vi "helperLoop.vi"(8 "error in (no error)":errorcluster, 11 "Connection Handler in":refnum<class "Connection Handler.lvclass">) -> (0 "error out":errorcluster, 3 "Connection Handler out":refnum<class "Connection Handler.lvclass">)   [LabVIEW 2017, in "Connection Handler.lvlib" / "Connection Handler.lvclass"]
uses:
  Connection Handler.lvclass
  Applications/National Instruments/LabVIEW 2017 64-bit/vi.lib/ActorFramework/Actor/Actor.lvclass
  Volumes/Data/Users/benji667/Git/BuildFarm/WebSocket Server/Actors/Actor wHelper/Actor wHelper/Actor wHelper.lvclass
  <vilib>/ActorFramework/Actor/Actor.lvclass/Actor.ctl
  <vilib>/ActorFramework/Message Enqueuer/Message Enqueuer.lvclass/Message Enqueuer.ctl
  Connection Handler.lvclass/Connection Handler.ctl
  Actor wHelper/Actor wHelper/Actor wHelper.lvclass/Actor wHelper.ctl
  Connection Handler Messages/Message Recieved Msg/Message Recieved Msg.lvclass/Message Recieved Msg.ctl
  Actor wHelper/Actor wHelper/Read StopHelperLoop Reg Ref.vi
  <vilib>/ActorFramework/Message Enqueuer/Init from Existing Queue.vi
  <vilib>/ActorFramework/Message Enqueuer/Enqueue.vi
  Connection Handler Messages/Message Recieved Msg/Message Recieved Msg.lvclass
  Applications/National Instruments/LabVIEW 2017 64-bit/vi.lib/ActorFramework/Message/Message.lvclass
  <vilib>/ActorFramework/Stop Msg/Stop Msg.lvclass
  <vilib>/ActorFramework/Message Priority Queue/Priority Enqueue.vi
  <vilib>/ActorFramework/Message Enqueuer/Message Enqueuer.lvclass
  Actor wHelper/Actor wHelper/Actor wHelper.lvclass
  <vilib>/MediaMongrels Ltd/WebSockets/Sockets/Socket/Socket.lvclass
  <vilib>/ActorFramework/Actor/Actor.lvclass
panel:
  out "Data":string
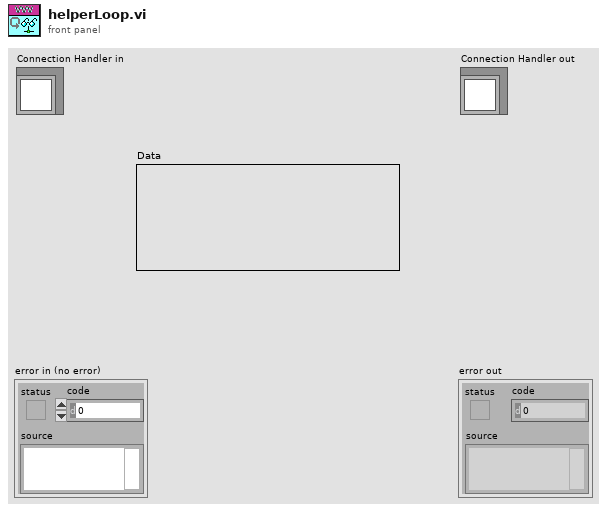
[diagram p1: front panel]
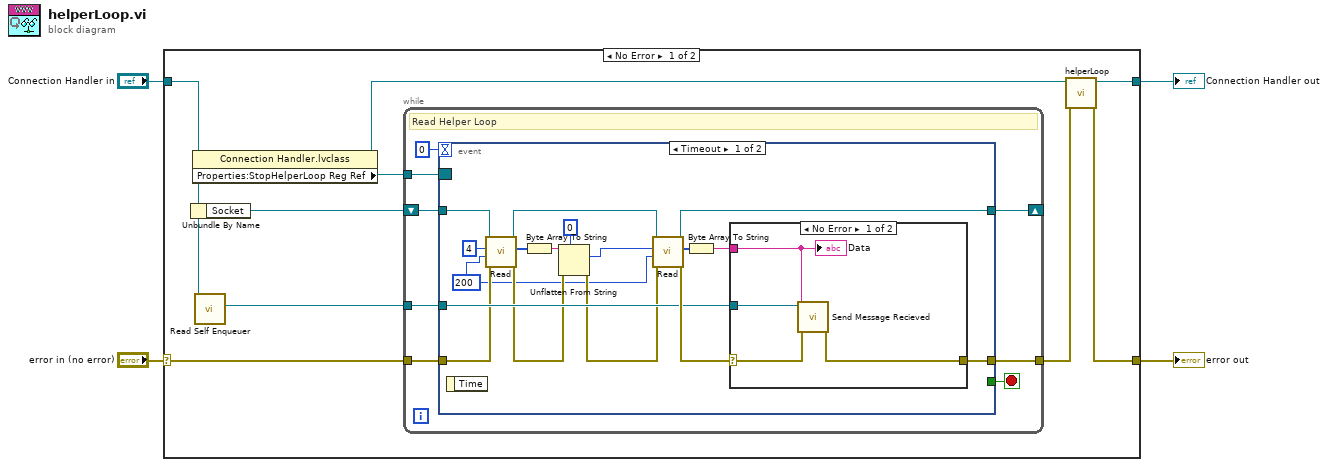
[diagram p0: block diagram]
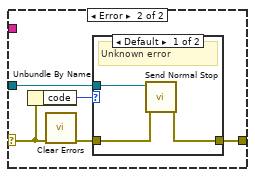
[diagram p2: hidden frame]
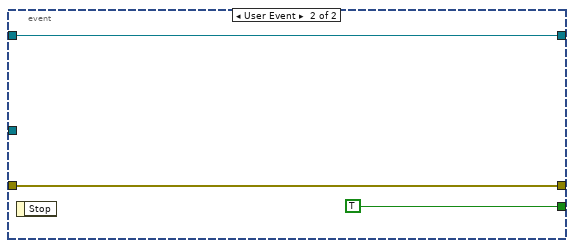
[diagram p4: hidden frame]
diagram:
  n1 = case shown="No Error" "error in (no error)" {
    selector: "error in (no error)" -> [w12 w56]
    tunnel: [w5 w56] -> w3
    tunnel: [w7 w55] -> w1
    tunnel: "Connection Handler in" -> [w10 w55]
    frame No Error {
      n2 = Unbundle By Name(w10) -> ("Socket"=w13:refnum<class "Socket.lvclass">)
      n3 = property class="Connection Handler.lvclass"(reference=w10) -> (reference out=w8:refnum<class "Connection Handler.lvclass">, "Properties:StopHelperLoop Reg Ref"=w9:refnum<event-registration>)  [unwired: 1 in, 1 out]
      n4 = call <vilib>:"Read Self Enqueuer.vi"("Actor"=w10) -> ("Self Enqueuer"=w11:refnum<class "Message Enqueuer.lvclass">)  [unwired: 10 in]
      n5 = while {
        tunnel: w9 -> [w21]
        tunnel: w11 -> [w18]
        shift-right: [w16] -> _
        shift-left: w13 -> [w19]
        tunnel: [w15] -> w6
        tunnel: w12 -> [w14]
        stop <- w20 stop-if-true
        # "Read Helper Loop"
        n6 = event shown="[0] Timeout" {
          selector: w21 -> [_ _]
          dyn-events: _ -> [_ _]
          timeout: 0 -> [_ _]
          tunnel: [_ TRUE] -> w20
          tunnel: w19 -> [w32 w53]
          tunnel: w18 -> [w34 _]
          tunnel: [w36 w53] -> w16
          tunnel: [w35 w52] -> w15
          tunnel: w14 -> [w23 w52]
          event Timeout {
            w22 = 200 ("timeout ms (5000)")
            n7 = event-data() -> ()  [unwired: 1 in, 1 out]
            n8 = call-dynamic "Read.vi"("error in (no error)"=w23, "timeout ms (25000)"=w22, "# bytes to read"=4, "Socket in"=w32) -> ("error out"=w25:errorcluster, "Read Bytes"=w29:u8[], "Socket out"=w31:refnum<class "Socket.lvclass">)  [unwired: 5 in]
            n9 = Byte Array To String(unsigned byte array=w29) -> (string=w28:string)
            n10 = Unflatten From String(type=0 ("bytes to read"), binary string=w28, error in (no error)=w25) -> (value=w26:i32, error out=w24:errorcluster)  [unwired: 1 in, 2 out]
            n11 = call-dynamic "Read.vi"("error in (no error)"=w24, "timeout ms (25000)"=w22, "# bytes to read"=w26, "Socket in"=w31) -> ("error out"=w38:errorcluster, "Read Bytes"=w37:u8[], "Socket out"=w36:refnum<class "Socket.lvclass">)  [unwired: 5 in]
            n12 = Byte Array To String(unsigned byte array=w37) -> (string=w33:string)
            n13 = case shown="No Error" w38 {
              selector: w38 -> [w41 w46]
              tunnel: w33 -> [w39 _]
              tunnel: w34 -> [w42 w45]
              tunnel: [w40 w43] -> w35
              frame No Error {
                n14 = call "Send Message Recieved.vi"("error in (no error)"=w41, "Message"=w39, "Message Enqueuer in"=w42) -> ("error out"=w40:errorcluster)  [unwired: 7 in, 1 out]
                "Data" <- w39
              }
              frame Error {
                n15 = Unbundle By Name(w46) -> ("code"=w47:i32)
                n16 = call <vilib>:"Clear Errors.vi"("error in (no error)"=w46) -> ("error out"=w44:errorcluster)  [unwired: 5 in, 1 out]
                n17 = case shown="Default" w47 {
                  tunnel: w44 -> [w48 w51]
                  tunnel: [w49 w51] -> w43
                  tunnel: w45 -> [w50 _]
                  frame Default {
                    # "Unknown error"
                    n18 = call <vilib>:"Send Normal Stop.vi"("error in (no error)"=w48, "Message Enqueuer"=w50) -> ("error out"=w49:errorcluster)  [unwired: 9 in]
                  }
                  frame 56 {
                    # "Ignore Timeout"
                  }
                }
              }
            }
          }
          event User Event {
            n19 = event-data() -> ()  [unwired: 1 in, 1 out]
          }
        }
      }
      n20 = call-parent "helperLoop.vi"("error in (no error)"=w6, "Actor wHelper in"=w8) -> ("error out"=w5:errorcluster, "Actor wHelper out"=w7:refnum<class "Connection Handler.lvclass">)  [unwired: 8 in]
    }
    frame Error {
    }
  }
  "error out" <- w3
  "Connection Handler out" <- w1
